vi "RSZVB Set Port Power Offset.vi"(6 "Port Power Offset (0)":dbl format="%^.3e", 7 "Offset Parameter (1: Add Channel Power)":i32(ring)=1 items=["Only", "Add Channel Power"], 8 "error in (no error)":errorcluster {"code" format="%.0x"}, 9 "Port Number (1)":i32=1, 10 "Channel (1)":i32=1, 11 "VISA session":refnum<visa-resource-name>) -> (0 "error out":errorcluster {"code" format="%.0x"}, 3 "dup VISA session":refnum<visa-resource-name>)   [LabVIEW 2011]
doc: "This VI defines a port-specific source power or a power offset relative to the channel power. \n\nRemote-control command(s):\nSOURce<Ch>:POWer<Pt>[:LEVel][:IMMediate]:OFFSet <numeric_value>, ONLY | CPADd"
uses:
  _utility/RSZVB Global Data.vi
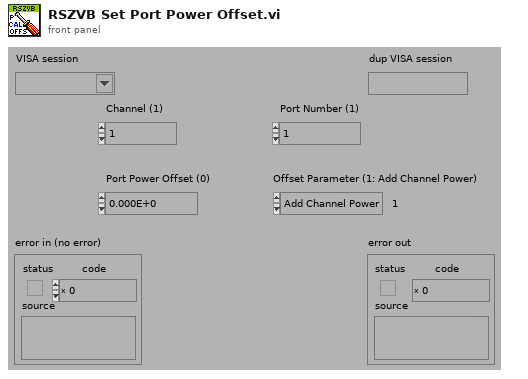
[diagram p1: front panel]
types:
  T1 = cluster{"Error Checking (T: On)":bool, "Installed Options":string[], "Data Valid?":bool, "Ports":i32, "Model":string[], "Option Checking (T: On)":bool}[]
  T2 = cluster{"Error Checking (T: On)":bool, "Installed Options":string[], "Data Valid?":bool, "Ports":i32, "Model":string[], "Option Checking (T: On)":bool}
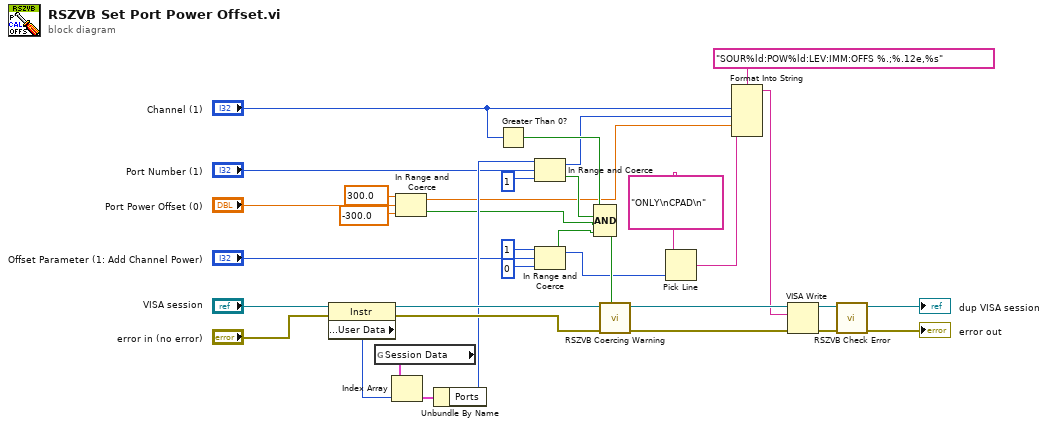
[diagram p0: block diagram]
diagram:
  n1 = property class="Instr"(reference="VISA session", error in="error in (no error)") -> (reference out=w21:refnum<visa-resource-name>, error out=w22:errorcluster, "General Settings:User Data"=w23:u32)
  n2 = global read "RSZVB Global Data.vi" "Session Data"() -> (w24:T1)
  n3 = Index Array(array=w24, index=w23) -> (element=w25:T2)
  n4 = In Range and Coerce(upper limit=300.0, x="Port Power Offset (0)", lower limit=-300.0) -> (coerced(x)=w2:dbl, In Range?=w3:bool)
  n5 = Unbundle By Name(w25) -> ("Ports"=w19:i32)
  n6 = Greater Than 0?(x="Channel (1)") -> (x > 0?=w26:bool)
  n7 = In Range and Coerce(upper limit=w19, x="Port Number (1)", lower limit=1) -> (coerced(x)=w17:i32, In Range?=w29:bool)
  n8 = In Range and Coerce(upper limit=1 ("lower limit"), x="Offset Parameter (1: Add Channel Power)", lower limit=0) -> (coerced(x)=w15:i32, In Range?=w14:bool)
  n9 = Compound Arithmetic op=AND(w26, w29, w3, w14) -> (w28:bool)
  n10 = call "RSZVB Coercing Warning.vi"("In Range?"=w28, "error in (no error)"=w22, "VISA session"=w21) -> ("error out"=w32:errorcluster, "dup VISA session"=w33:refnum<visa-resource-name>)  [unwired: 7 in]
  n11 = Pick Line(multi-line string="ONLY\nCPAD\n", line index=w15) -> (output string=w13:string)  [unwired: 1 in]
  n12 = Format Into String(format string="SOUR%ld:POW%ld:LEV:IMM:OFFS %.;%.12e,%s", "Channel (1)", w17, w2, w13) -> (resulting string=w27:string)  [unwired: 2 in, 1 out]
  n13 = VISA Write(VISA resource name=w33, write buffer=w27, error in (no error)=w32) -> (VISA resource name out=w30:refnum<visa-resource-name>, error out=w31:errorcluster)  [unwired: 1 out]
  n14 = call "RSZVB Check Error.vi"("error in (no error)"=w31, "VISA session"=w30) -> ("error out"=→"error out":errorcluster, "dup VISA session"=→"dup VISA session":refnum<visa-resource-name>)  [unwired: 8 in]
